vi "Get Data.vi"(8 "error in (no error)":errorcluster, 11 "Pulse Recorder in":refnum<class "Pulse Recorder.lvclass">) -> (0 "error out":errorcluster, 2 "Data Result":refnum<class "Acquired Result.lvclass">, 3 "Pulse Recorder out":refnum<class "Pulse Recorder.lvclass">)   [LabVIEW 2015, in "Pulse Recorder.lvclass"]
uses:
  Pulse Recorder.lvclass
  NHMFL_Core/Libraries/Instruments/Pulse Driver/Pulse Driver.lvclass
  Results/Acquired Result/Acquired Result.lvclass
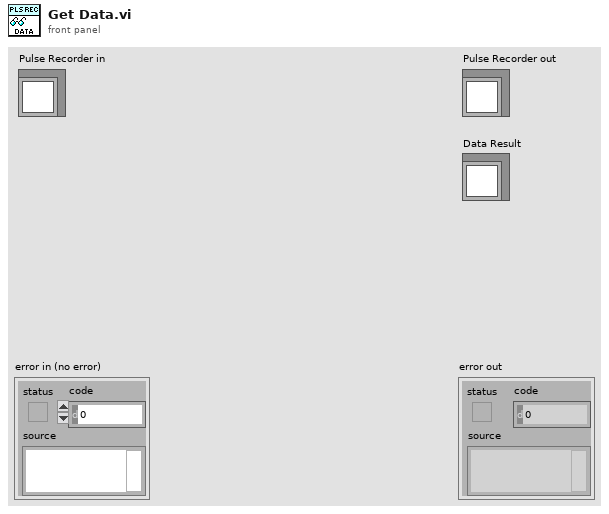
[diagram p1: front panel]
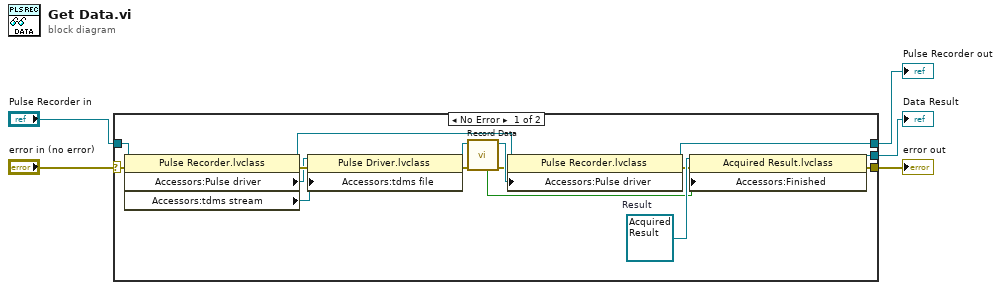
[diagram p0: block diagram]
diagram:
  n1 = case shown="No Error" "error in (no error)" {
    selector: "error in (no error)" -> [w13 w23]
    tunnel: [w8 w23] -> w4
    tunnel: [w11 w22] -> w2
    tunnel: "Pulse Recorder in" -> [w12 w22]
    tunnel: [w7 _] -> w1
    frame No Error {
      w10 = refnum<class "Acquired Result.lvclass"> refnum  # Result
      n2 = property class="Pulse Recorder.lvclass"(reference=w12, error in=w13) -> (reference out=w21:refnum<class "Pulse Recorder.lvclass">, error out=w20:errorcluster, "Accessors:Pulse driver"=w19:refnum<class "Pulse Driver.lvclass">, "Accessors:tdms stream"=w18:refnum<k34>)
      n3 = property class="Pulse Driver.lvclass"(reference=w19, error in=w20, "Accessors:tdms file"=w18) -> (reference out=w17:refnum<class "Pulse Driver.lvclass">, error out=w15:errorcluster)
      n4 = call-dynamic "Record Data.vi"("error in (no error)"=w15, "Pulse Driver in"=w17) -> ("error out"=w14:errorcluster, "Pulse Driver out"=w16:refnum<class "Pulse Driver.lvclass">, "Finished"=w6:bool)  [unwired: 7 in]
      n5 = property class="Pulse Recorder.lvclass"(reference=w21, error in=w14, "Accessors:Pulse driver"=w16) -> (reference out=w11:refnum<class "Pulse Recorder.lvclass">, error out=w9:errorcluster)
      n6 = property class="Acquired Result.lvclass"(reference=w10, error in=w9, "Accessors:Finished"=w6) -> (reference out=w7:refnum<class "Acquired Result.lvclass">, error out=w8:errorcluster)
    }
    frame Error {
    }
  }
  "error out" <- w4
  "Pulse Recorder out" <- w2
  "Data Result" <- w1
